vi "U6 CR Speed Test.vi"() -> ()   [LabVIEW 2021]
panel:
  in  "Enable Interval Timing":bool
  out "min ms":u32
  out "max ms":u32
  out "avg ms per iteration":dbl format="%.2f"
  out "Array":u32[](array[numeric])
  in  "Write Both DACs":bool
  in  "Write Digital":bool
  in  "Read Digital":bool
  out "total ms":u32
  in  "AIN Range":string="LJ_rgBIP10V"
  in  "# Iterations":i32=128
  in  "# AIN Channels":i32=1
  in  "SettlingFactor":i32
  out "Error Message":string
  in  "Resolution":i32=8
  out "error out":errorcluster
  # "Aquires multiple analog input channels over USB from the first found U6."
  # "LJ_rgBIP10V\nLJ_rgBIP1V\nLJ_rgBIPP1V\nLJ_rgBIPP01V"
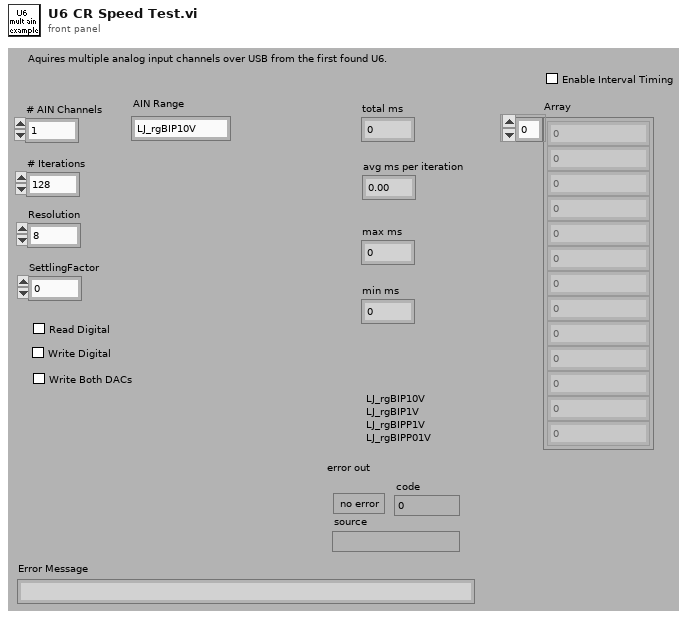
[diagram p1: front panel]
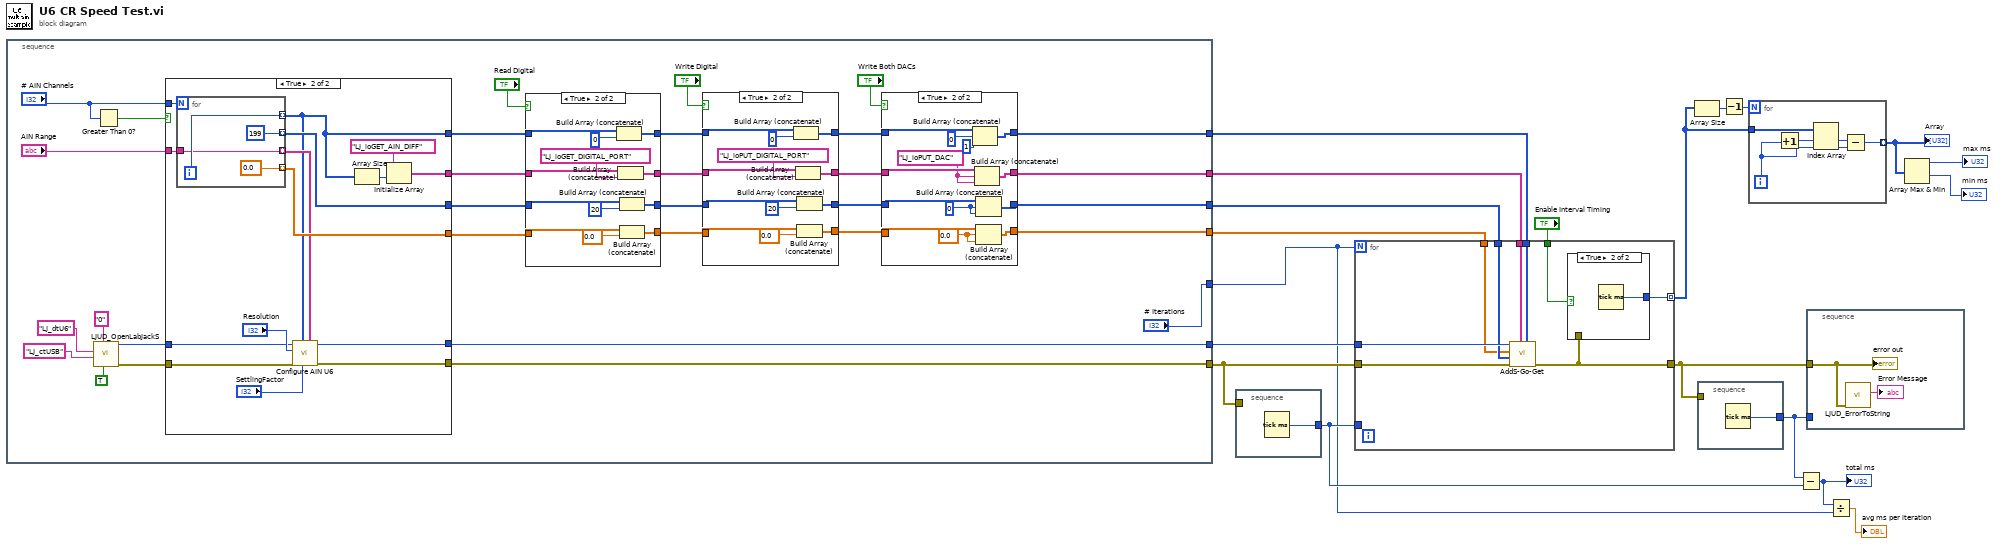
[diagram p0: block diagram]
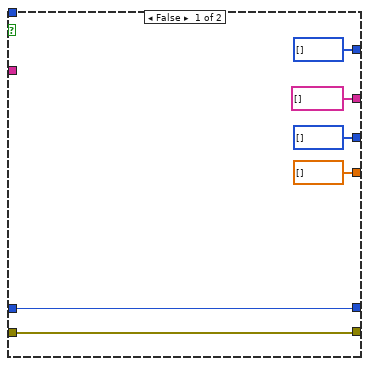
[diagram p2: hidden frame]
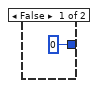
[diagram p6: hidden frame]
diagram:
  n1 = stacked-sequence {
    tunnel: [w20] -> w19
    tunnel: [w22] -> w15
    tunnel: [w31] -> w18
    tunnel: [w32] -> w17
    tunnel: [w30] -> w16
    tunnel: ["# Iterations"] -> w5
    tunnel: [w29] -> w11
    frame #0 {
      n2 = call "LJUD_OpenLabJackS.vi"("FirstFound"=TRUE, "Address"="0", "ConnectionType"="LJ_ctUSB", "DeviceType"="LJ_dtU6") -> ("error out"=w23:errorcluster, "Handle"=w21:i32)  [unwired: 5 in, 1 out]
      n3 = Greater Than 0?(x="# AIN Channels") -> (x > 0?=w25:bool)
      n4 = case shown="True" w25 {
        tunnel: "# AIN Channels" -> [_ w69]
        tunnel: "AIN Range" -> [_ w68]
        tunnel: [string[] [] w67] -> w44
        tunnel: [i32[] [] w66] -> w43
        tunnel: [dbl[] [] w65] -> w42
        tunnel: [i32[] [] w57] -> w24
        tunnel: w23 -> [w51 w62]
        tunnel: [w51 w61] -> w22
        tunnel: w21 -> [w52 w60]
        tunnel: [w52 w59] -> w20
        frame False {
        }
        frame True {
          n5 = for {
            N: w69 -> [_]
            tunnel: [w75] -> w57 mode=indexing
            tunnel: [w74] -> w58 mode=indexing
            tunnel: w68 -> [w74]
            tunnel: [199] -> w66 mode=indexing
            tunnel: [0.0] -> w65 mode=indexing
            i -> [w75]
          }
          n6 = call "Configure AIN U6.vi"("Ranges"=w58, "SettlingFactor"="SettlingFactor", "Positive Channels"=w57, "error in"=w62, "Resolution"="Resolution", "Handle In"=w60) -> ("error out"=w61:errorcluster, "Handle Out"=w59:i32)  [unwired: 4 in]
          n7 = Array Size(array=w57) -> (size(s)=w71:i32)
          n8 = Initialize Array("LJ_ioGET_AIN_DIFF" ("IOType"), w71) -> (w67:string[])
        }
      }
      n9 = case shown="True" "Read Digital" {
        tunnel: [w112 w124] -> w40
        tunnel: w24 -> [w112 w118]
        tunnel: [w111 w123] -> w39
        tunnel: w44 -> [w111 w121]
        tunnel: [w110 w115] -> w38
        tunnel: w43 -> [w110 w120]
        tunnel: w42 -> [w109 w114]
        tunnel: [w109 w113] -> w37
        frame False {
        }
        frame True {
          n10 = Build Array (concatenate)(w118, 0) -> (w124:i32[])
          n11 = Build Array (concatenate)(w121, "LJ_ioGET_DIGITAL_PORT" ("IOType")) -> (w123:string[])
          n12 = Build Array (concatenate)(w120, 20) -> (w115:i32[])
          n13 = Build Array (concatenate)(w114, 0.0) -> (w113:dbl[])
        }
      }
      n14 = case shown="True" "Write Digital" {
        tunnel: [w96 w108] -> w36
        tunnel: w40 -> [w96 w102]
        tunnel: [w95 w107] -> w35
        tunnel: w39 -> [w95 w105]
        tunnel: [w94 w99] -> w34
        tunnel: w38 -> [w94 w104]
        tunnel: w37 -> [w93 w98]
        tunnel: [w93 w97] -> w33
        frame False {
        }
        frame True {
          n15 = Build Array (concatenate)(w102, 0) -> (w108:i32[])
          n16 = Build Array (concatenate)(w105, "LJ_ioPUT_DIGITAL_PORT" ("IOType")) -> (w107:string[])
          n17 = Build Array (concatenate)(w104, 20) -> (w99:i32[])
          n18 = Build Array (concatenate)(w98, 0.0) -> (w97:dbl[])
        }
      }
      n19 = case shown="True" "Write Both DACs" {
        tunnel: [w79 w92] -> w32
        tunnel: w36 -> [w79 w88]
        tunnel: [w78 w91] -> w31
        tunnel: w35 -> [w78 w90]
        tunnel: [w77 w87] -> w30
        tunnel: w34 -> [w77 w89]
        tunnel: w33 -> [w76 w86]
        tunnel: [w76 w85] -> w29
        frame False {
        }
        frame True {
          w84 = "LJ_ioPUT_DAC" ("IOType")
          w82 = 0.0
          w83 = 0
          n20 = Build Array (concatenate)(w88, 0, 1) -> (w92:i32[])
          n21 = Build Array (concatenate)(w90, w84, w84) -> (w91:string[])
          n22 = Build Array (concatenate)(w89, w83, w83) -> (w87:i32[])
          n23 = Build Array (concatenate)(w86, w82, w82) -> (w85:dbl[])
        }
      }
    }
  }
  n24 = stacked-sequence {
    tunnel: w15 -> [_]
    tunnel: [w125] -> w12
    frame #0 {
      n25 = Tick Count (ms)() -> (millisecond timer value=w125:u32)
    }
  }
  n26 = for {
    N: w5 -> [_]
    tunnel: w19 -> [w134]
    tunnel: w15 -> [w133]
    tunnel: [w127] -> w14
    tunnel: w18 -> [w132]
    tunnel: w17 -> [w131]
    tunnel: w16 -> [w130]
    tunnel: w12 -> [_]
    tunnel: w11 -> [w129]
    tunnel: "Enable Interval Timing" -> [w128]
    tunnel: [w126] -> w4 mode=indexing
    n27 = call "AddS-Go-Get.vi"("Channels"=w131, "IOTypes"=w132, "error in"=w133, "x1"=w130, "Values Write"=w129, "Handle In"=w134) -> ("error out"=w127:errorcluster)  [unwired: 3 in, 2 out]
    n28 = case shown="True" w128 {
      tunnel: w127 -> [_ _]
      tunnel: [u32 0 ("millisecond timer value") w136] -> w126
      frame False {
      }
      frame True {
        n29 = Tick Count (ms)() -> (millisecond timer value=w136:u32)
      }
    }
  }
  n30 = Array Size(array=w4) -> (size(s)=w9:i32)
  n31 = stacked-sequence {
    tunnel: w14 -> [_]
    tunnel: [w137] -> w13
    frame #0 {
      n32 = Tick Count (ms)() -> (millisecond timer value=w137:u32)
    }
  }
  n33 = Decrement(x=w9) -> (x-1=w8:i32)
  n34 = for {
    N: w8 -> [_]
    tunnel: w4 -> [w143]
    tunnel: [w138] -> w3 mode=indexing
    i -> [w141]
    n35 = Increment(x=w141) -> (x+1=w142:i32)
    n36 = Index Array(array=w143, index #1=w142, index #2=w141) -> (element #1=w139:u32, element #2=w140:u32)
    n37 = Subtract(x=w139, y=w140) -> (x-y=w138:u32)
  }
  "Array" <- w3
  n38 = Subtract(x=w13, y=w12) -> (x-y=w6:u32)
  "total ms" <- w6
  n39 = stacked-sequence {
    tunnel: w14 -> [w144]
    tunnel: w13 -> [_]
    frame #0 {
      n40 = call "LJUD_ErrorToString.vi"("error in"=w144) -> ("String"=→"Error Message":string)  [unwired: 10 in]
      "error out" <- w144
    }
  }
  n41 = Divide(x=w6, y=w5) -> (x/y=→"avg ms per iteration":dbl)
  n42 = Array Max & Min(array=w3) -> (max value=→"max ms":u32, min value=→"min ms":u32)  [unwired: 2 out]
